vi "TestStand_Go to Temperature Setpoint.vi"(5 "Soak (s)":u32=180, 7 "Timeout (s)":u32=120, 9 "PID Parameters":T1={"Proportional"=0.05, "Integral"=0.0005, "Differential"=-0.0005}, 10 "Tolerance":dbl=0.25 format="%.2f", 11 "Temperature Target":dbl=37.5 caption="Target" format="%.2f") -> (0 "Error Out":errorcluster, 1 "RTD1 Temperature (°C)":dbl=nan format="%.2f", 2 "UUT Temperature (°C)":dbl=nan format="%.2f", 3 "Final Setpoint":dbl=nan format="%.2f", 4 "xPG Charging State":string, 6 "xPG Temperature Level":dbl=nan, 8 "IPG_ReceivedLevel":dbl=nan)   [LabVIEW 2010]
uses:
  Calculations/Temperature Setpoint States.ctl
  <vilib>/ptbypt/NI_PtbyPt.lvlib
panel:
  out "Raw Corrected Temp (°C)":dbl
  in  "stop":bool
  out "Temperature and Delta History":T2(graph)
  out "Setpoint (°C)":dbl=nan format="%.2g"
  out "Temperature Target (°C)":dbl=nan min=25.0 max=80.0 step=0.1 format="%.2f"
  out "Delta_IPG_Target (°C)":dbl=nan format="%.2f"
  out "Air Temperature (°C)":dbl=nan min=25.0 max=80.0 step=0.1 format="%.2f"
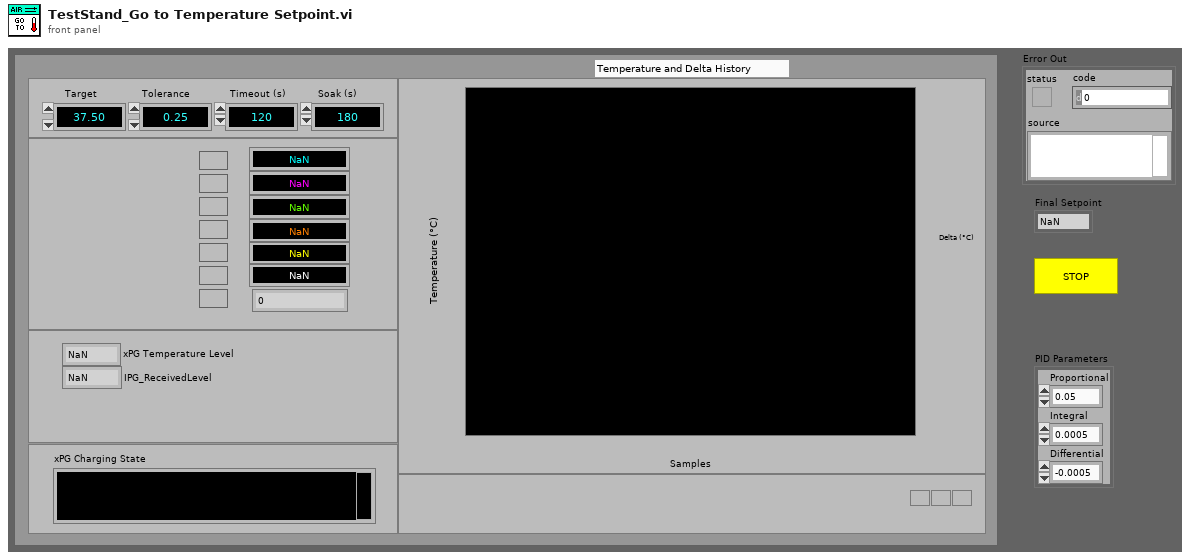
[diagram p1: front panel]
types:
  T1 = cluster{"Proportional":dbl, "Integral":dbl, "Differential":dbl}
  T2 = cluster{"Temperature Target":dbl, "Air Temperature (°C)":dbl, "UUT Temperature (°C)":dbl, "RTD1 Temperature (°C)":dbl, "Setpoint (°C)":dbl, "Delta Setpoint (°C)":dbl, "Delta Setpoint (°C) 2":dbl}
  T3 = cluster{"Temperature Target":dbl, "Air Temperature (°C)":dbl, "UUT Temperature (°C)":dbl, "RTD1 Temperature (°C)":dbl, "Setpoint (°C)":dbl, "Delta Setpoint (°C)":dbl, "Raw Corrected Temp (°C)":dbl}
  T4 = cluster{"Data Index":i32, "Air Blast Ref":refnum<visa-resource-name>, "Tolerance":dbl, "Timeout At":timestamp, "Timed out?":bool, "Previous Millis":u32, "Init PI?":bool, "Soaking?":bool, "Soak Finished At":timestamp, "PID Parameters":cluster{"Proportional":dbl, "Integral":dbl, "Differential":dbl}, "Blast Mode?":bool, "Soak Time (s)":u32, "Init Filter":bool}
  T5 = typedef "Temperature Setpoint States.ctl" = enum16{"Initialize", "Measure", "Update Setpoint", "Update Display", "Check If Done"}
  T6 = cluster{"Temperature Target":dbl, "Air Temperature (°C)":dbl, "UUT Temperature (°C)":dbl, "RTD Temperature (°C)":dbl, "Delta Setpoint (°C)":dbl, "Setpoint (°C)":dbl, "Setpoint (°C) 2":dbl}[]
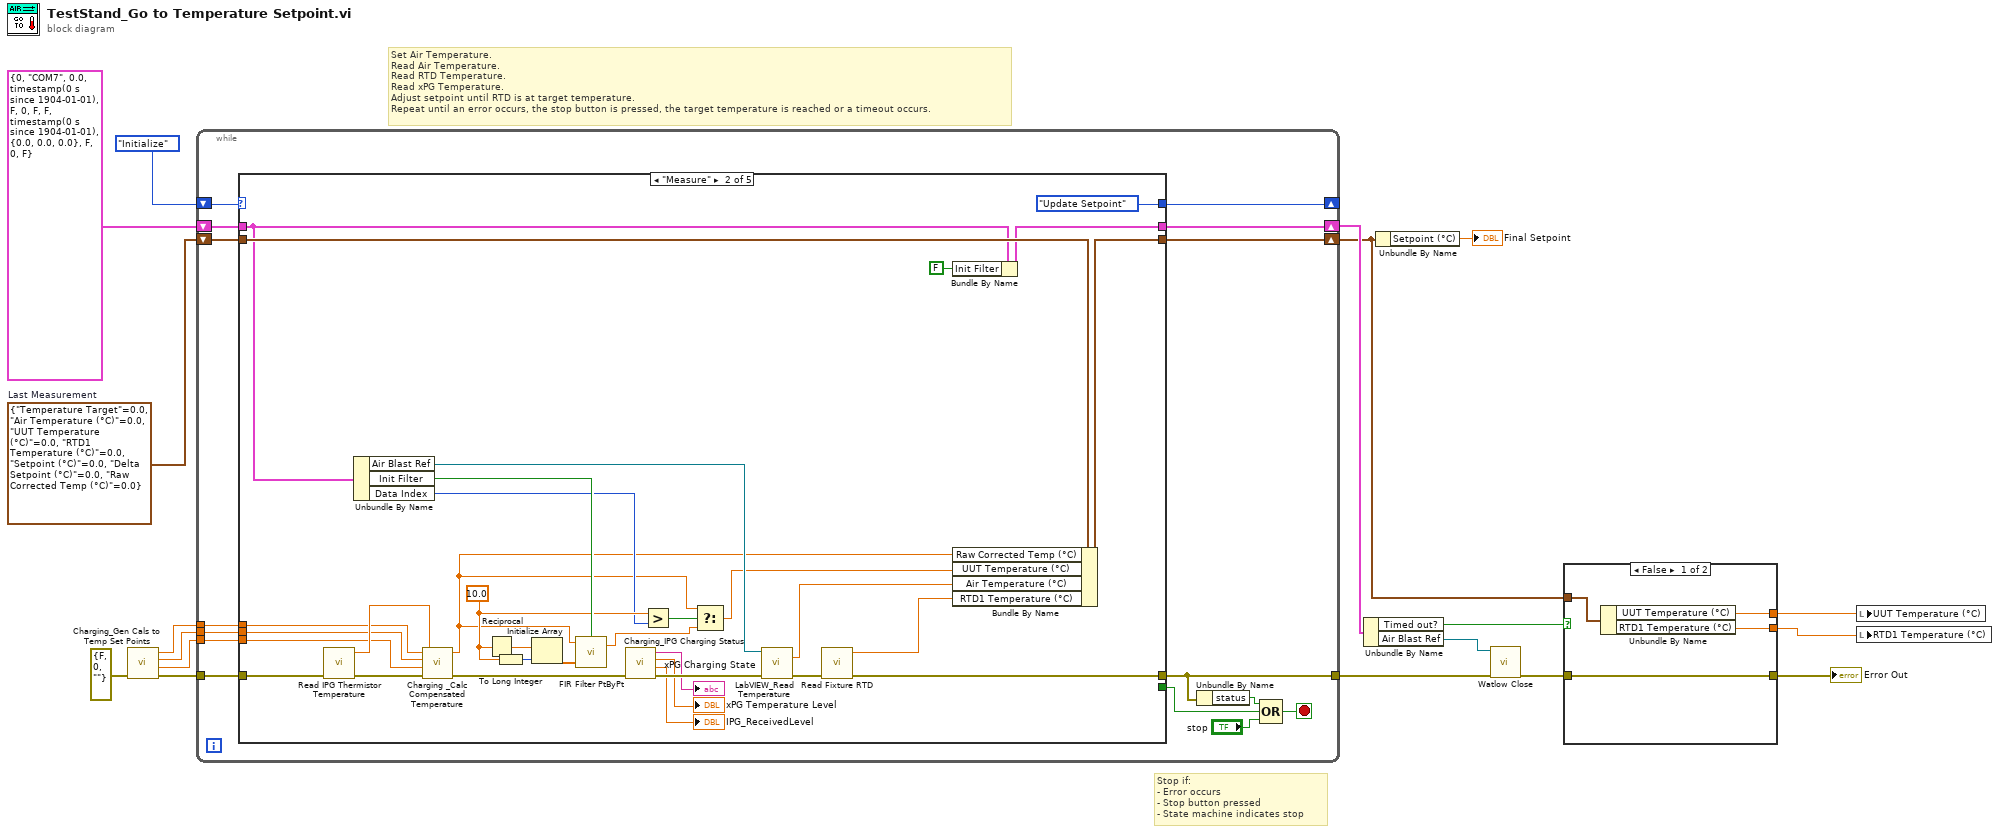
[diagram p0: block diagram]
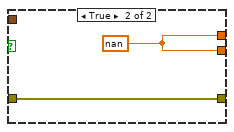
[diagram p2: hidden frame]
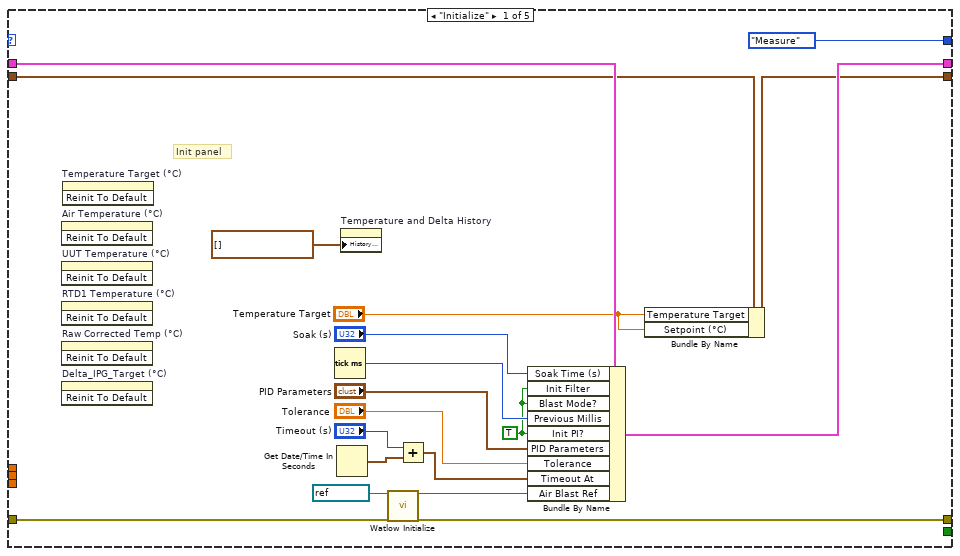
[diagram p3: hidden frame]
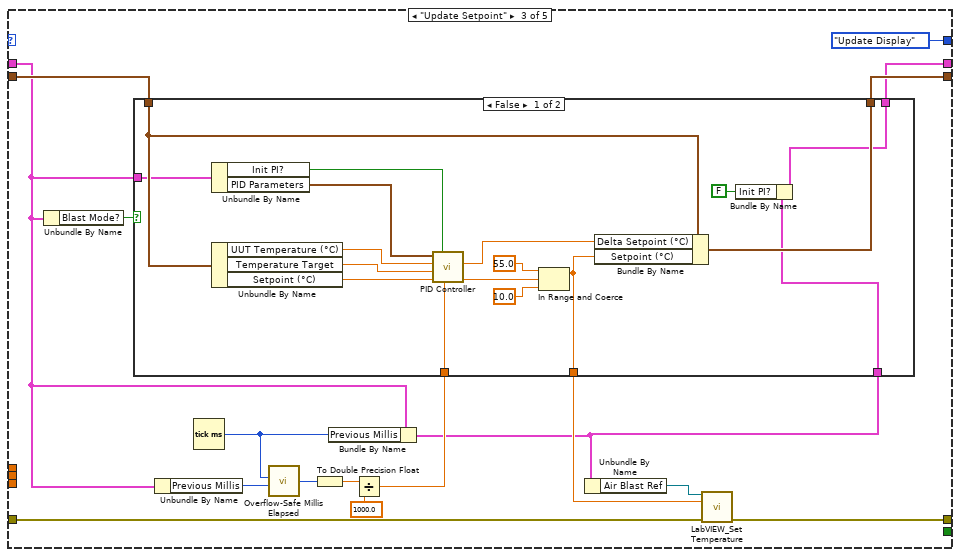
[diagram p4: hidden frame]
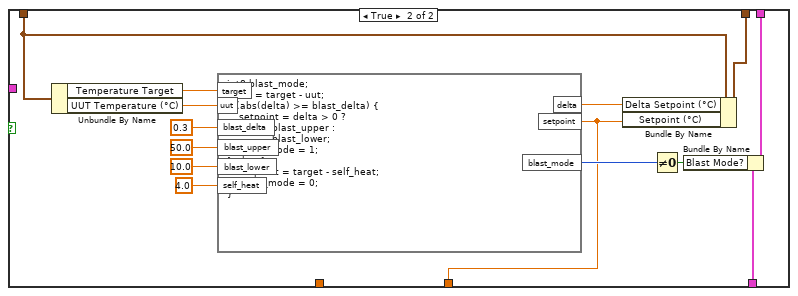
[diagram p5: hidden frame]
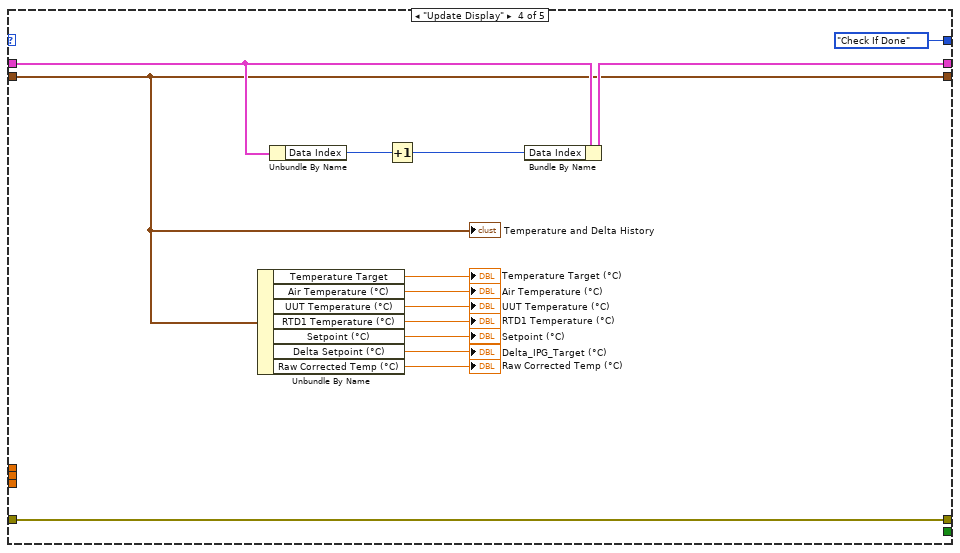
[diagram p6: hidden frame]
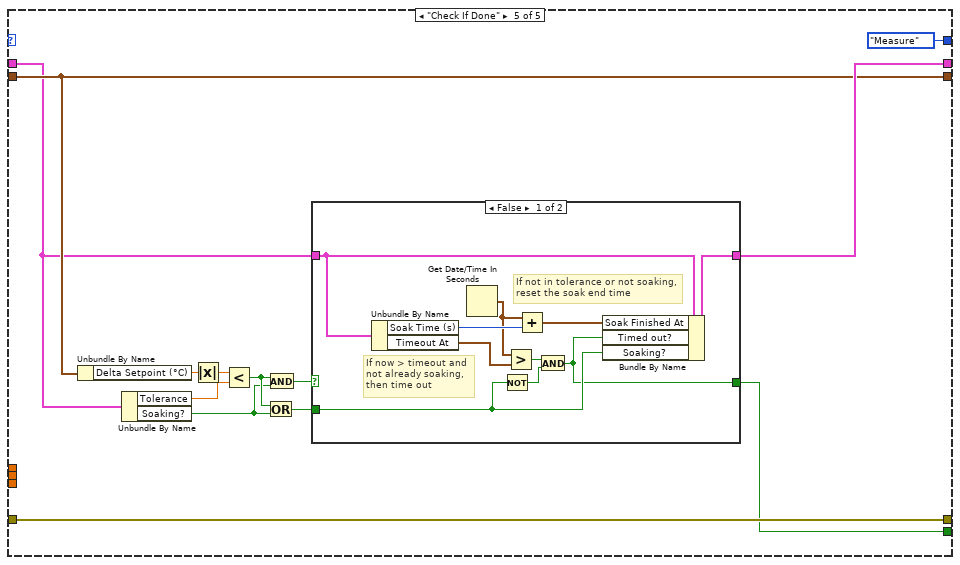
[diagram p7: hidden frame]
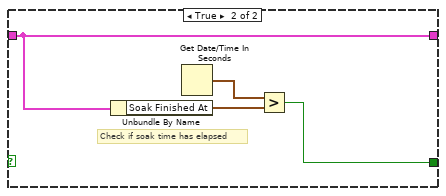
[diagram p8: hidden frame]
diagram:
  w16 = T3 {"Temperature Target"=0.0, "Air Temperature (°C)"=0.0, "UUT Temperature (°C)"=0.0, "RTD1 Temperature (°C)"=0.0, "Setpoint (°C)"=0.0, "Delta Setpoint (°C)"=0.0, "Raw Corrected Temp (°C)"=0.0}  # Last Measurement
  # "Set Air Temperature.\nRead Air Temperature.\nRead RTD Temperature.\nRead xPG Temperature.\nAdjust setpoint until RTD is at target temperature.\nRepeat until an error occurs, the stop button is pressed, the target temperature is reached or a timeout occurs."
  # "Stop if:\n- Error occurs\n- Stop button pressed\n- State machine indicates stop"
  n1 = call "Charging_Gen Cals to Temp Set Points.vi"("error in"=errorcluster {"status"=FALSE, "code"=0, "source"=""} ("Error Out")) -> ("error out"=w10:errorcluster, "Abort Threshold (C)"=w7:dbl, "Critical Threshold (C)"=w8:dbl, "Warning Threshold (C)"=w9:dbl)  [unwired: 6 in, 1 out]
  n2 = while {
    shift-right: [w22] -> _
    shift-left: Temperature_Setpoint_States."Initialize" ("Temperature Setpoint States") -> [w33]
    shift-right: [w32] -> w13
    shift-left: T4 {"Data Index"=0, "Air Blast Ref"="COM7", "Tolerance"=0.0, "Timeout At"=timestamp(0 s since 1904-01-01), "Timed out?"=FALSE, "Previous Millis"=0, "Init PI?"=FALSE, "Soaking?"=FALSE, "Soak Finished At"=timestamp(0 s since 1904-01-01), "PID Parameters"={"Proportional"=0.0, "Integral"=0.0, "Differential"=0.0}, "Blast Mode?"=FALSE, "Soak Time (s)"=0, "Init Filter"=FALSE} -> [w31]
    shift-right: [w23] -> w3
    shift-left: w16 -> [w30]
    tunnel: [w27] -> w14
    tunnel: w10 -> [w29]
    tunnel: w9 -> [w21]
    tunnel: w8 -> [w20]
    tunnel: w7 -> [w19]
    stop <- w28 stop-if-true
    n3 = case shown="\"Measure\"" w33 {
      tunnel: [_ _ _ _ w156] -> w25
      tunnel: [Temperature_Setpoint_States."Measure" ("Temperature Setpoint States") Temperature_Setpoint_States."Update Setpoint" ("Temperature Setpoint States") Temperature_Setpoint_States."Update Display" ("Temperature Setpoint States") Temperature_Setpoint_States."Check If Done" ("Temperature Setpoint States") Temperature_Setpoint_States."Measure" ("Temperature Setpoint States")] -> w22
      tunnel: [w48 w65 w86 w143 w157] -> w32
      tunnel: w31 -> [w50 w66 w88 w145 w151]
      tunnel: w30 -> [w40 w80 w95 w134 w152]
      tunnel: w29 -> [w46 w83 w94 w138 w159]
      tunnel: [w45 w77 w90 w138 w159] -> w27
      tunnel: [w39 w78 w91 w134 w152] -> w23
      tunnel: w21 -> [_ w73 _ _ _]
      tunnel: w20 -> [_ w72 _ _ _]
      tunnel: w19 -> [_ w71 _ _ _]
      frame "Initialize" {
        w35 = TRUE ("Init PID?")
        # "Init panel"
        n4 = invoke on="Air Temperature (°C)" class="DigNum (strict)" method="Reinit To Default"() -> ()  [unwired: 3 in, 3 out]
        n5 = invoke on="UUT Temperature (°C)" class="DigNum (strict)" method="Reinit To Default"() -> ()  [unwired: 3 in, 3 out]
        n6 = invoke on="RTD1 Temperature (°C)" class="DigNum (strict)" method="Reinit To Default"() -> ()  [unwired: 3 in, 3 out]
        n7 = invoke on="Raw Corrected Temp (°C)" class="DigNum (strict)" method="Reinit To Default"() -> ()  [unwired: 3 in, 3 out]
        n8 = invoke on="Delta_IPG_Target (°C)" class="DigNum (strict)" method="Reinit To Default"() -> ()  [unwired: 3 in, 3 out]
        n9 = invoke on="Temperature Target (°C)" class="DigNum (strict)" method="Reinit To Default"() -> ()  [unwired: 3 in, 3 out]
        n10 = Tick Count (ms)() -> (millisecond timer value=w37:u32)
        n11 = Get Date/Time In Seconds() -> (seconds since 1Jan1904=w47:timestamp)
        n12 = property on="Temperature and Delta History" class="WFChart (strict)"("History Data"=T6 []) -> ()  [unwired: 2 in, 2 out]
        n13 = call <instrlib>:"Watlow Initialize.vi"("Comms Port"=refnum<visa-resource-name> "COM7", "Error In"=w46) -> ("UUT Port 2"=w49:refnum<visa-resource-name>, "Error Out"=w45:errorcluster)  [unwired: 16 out]
        n14 = Add(x="Timeout (s)", y=w47) -> (x+y=w43:timestamp)
        n15 = Bundle By Name(cluster=w50, "Soak Time (s)"="Soak (s)", "Init Filter"=w35, "Blast Mode?"=w35, "Previous Millis"=w37, "Init PI?"=w35, "PID Parameters"="PID Parameters", "Tolerance"="Tolerance", "Timeout At"=w43, "Air Blast Ref"=w49) -> (w48:T4)
        n16 = Bundle By Name(cluster=w40, "Temperature Target"="Temperature Target", "Setpoint (°C)"="Temperature Target") -> (w39:T3)
      }
      frame "Measure" {
        w63 = 10.0
        n17 = call "Read IPG Thermistor Temperature.vi"("error in"=w83) -> ("error out"=w74:errorcluster, "Compensated Temperature (C)"=w75:dbl)  [unwired: 7 in, 2 out]
        n18 = Unbundle By Name(w66) -> ("Air Blast Ref"=w82:refnum<visa-resource-name>, "Init Filter"=w67:bool, "Data Index"=w59:i32)
        n19 = call "Charging _Calc Compensated Temperature.vi"("target temperature (C)"=w75, "error in"=w74, "Abort Threshold (42 C)"=w71, "Critical Threshold (41 C)"=w72, "Warning Threshold (40 C)"=w73) -> ("error out"=w58:errorcluster, "compensated temperature (C)"=w53:dbl)  [unwired: 2 in, 1 out]
        n20 = Reciprocal(x=w63) -> (1/x=w70:dbl)
        n21 = To Long Integer(number=w63) -> (32bit integer=w69:i32)
        n22 = Initialize Array(w70, w69) -> (w68:dbl[])
        n23 = call <vilib>:"FIR Filter PtByPt.vi"("initialize"=w67, "Forward Coefficients"=w68, "x"=w53) -> ("Filtered x"=w60:dbl)  [unwired: 1 in, 1 out]
        n24 = call "Charging_IPG Charging Status.vi"("error in"=w58) -> ("error out"=w57:errorcluster, "IPG_ReceivedLevel"=→"IPG_ReceivedLevel":dbl, "TemperatureLevel"=→"xPG Temperature Level":dbl, "ChargingState"=→"xPG Charging State":string)  [unwired: 7 in]
        n25 = Greater?(x=w63, y=w59) -> (0:w62:bool)
        n26 = Select(t=w53, s=w62, f=w60) -> (s? t:f=w61:dbl)
        n27 = call "LabVIEW_Read Temperature.vi"("PC Comms Port"=w82, "error in (no error)"=w57) -> ("Air Temperature (°C)"=w81:dbl, "error out"=w84:errorcluster)  [unwired: 11 in, 1 out]
        n28 = call "Read Fixture RTD.vi"("error in (no error)"=w84) -> ("error out"=w77:errorcluster, "Mean Temperature (C)"=w79:dbl)  [unwired: 7 in, 1 out]
        n29 = Bundle By Name(cluster=w66, "Init Filter"=FALSE) -> (w65:T4)
        n30 = Bundle By Name(cluster=w80, "Raw Corrected Temp (°C)"=w53, "UUT Temperature (°C)"=w61, "Air Temperature (°C)"=w81, "RTD1 Temperature (°C)"=w79) -> (w78:T3)
      }
      frame "Update Setpoint" {
        n31 = Unbundle By Name(w88) -> ("Blast Mode?"=w87:bool)
        n32 = Unbundle By Name(w88) -> ("Previous Millis"=w98:u32)
        n33 = Tick Count (ms)() -> (millisecond timer value=w97:u32)
        n34 = call "Overflow-Safe Millis Elapsed.vi"("now"=w97, "previous"=w98) -> ("elapsed"=w101:u32)  [unwired: 5 in]
        n35 = To Double Precision Float(number=w101) -> (double precision float=w99:dbl)
        n36 = Bundle By Name(cluster=w88, "Previous Millis"=w97) -> (w85:T4)
        n37 = Divide(x=w99, y=1000.0) -> (x/y=w96:dbl)
        n38 = case shown="False" w87 {
          tunnel: w96 -> [w118 _]
          tunnel: w95 -> [w117 w121]
          tunnel: [w116 w119] -> w93
          tunnel: [w115 w120] -> w91
          tunnel: w88 -> [w107 _]
          tunnel: [w103 w131] -> w86
          tunnel: w85 -> [w102 w132]
          frame False {
            n39 = Unbundle By Name(w107) -> ("Init PI?"=w106:bool, "PID Parameters"=w105:T1)
            n40 = Unbundle By Name(w117) -> ("UUT Temperature (°C)"=w109:dbl, "Temperature Target"=w110:dbl, "Setpoint (°C)"=w111:dbl)
            n41 = call "PID Controller.vi"("dt"=w118, "Initialize"=w106, "Previous Set Point"=w111, "Desired Setpoint"=w110, "Measured"=w109, "PID Parameters"=w105) -> ("New Setpoint"=w112:dbl, "Error"=w108:dbl)  [unwired: 4 in]
            n42 = In Range and Coerce(upper limit=55.0 ("y"), x=w112, lower limit=10.0 ("y")) -> (coerced(x)=w116:dbl)  [unwired: 1 out]
            n43 = Bundle By Name(cluster=w117, "Delta Setpoint (°C)"=w108, "Setpoint (°C)"=w116) -> (w115:T3)
            n44 = Bundle By Name(cluster=w102, "Init PI?"=FALSE) -> (w103:T4)
          }
          frame True {
            n45 = Unbundle By Name(w121) -> ("Temperature Target"=w128:dbl, "UUT Temperature (°C)"=w127:dbl)
            n46 = formula code="int8 blast_mode;\ndelta = target - uut;\nif (abs(delta) >= blast_delta) {\n    setpoint = delta > 0 ? \n               blast_upper :\n               blast_lower;\n    blast_mode = 1;\n} else {\n    setpoint = target - self_heat;\n    blast_mode = 0;\n}"("target"=w128, "uut"=w127, "self_heat"=4.0 ("input variable"), "blast_delta"=0.3 ("input variable"), "blast_upper"=50.0 ("input variable"), "blast_lower"=10.0 ("input variable")) -> ("delta"=w122:dbl, "setpoint"=w119:dbl, "blast_mode"=w130:i8)
            n47 = Bundle By Name(cluster=w121, "Delta Setpoint (°C)"=w122, "Setpoint (°C)"=w119) -> (w120:T3)
            n48 = Not Equal To 0?(x=w130) -> (x != 0?=w129:bool)
            n49 = Bundle By Name(cluster=w132, "Blast Mode?"=w129) -> (w131:T4)
          }
        }
        n50 = Unbundle By Name(w85) -> ("Air Blast Ref"=w92:refnum<visa-resource-name>)
        n51 = call "LabVIEW_Set Temperature.vi"("PC Comms Port"=w92, "Air Temperature Setpoint (°C)"=w93, "error in (no error)"=w94) -> ("error out"=w90:errorcluster)  [unwired: 11 in, 1 out]
      }
      frame "Update Display" {
        n52 = Unbundle By Name(w134) -> ("Temperature Target"=→"Temperature Target (°C)":dbl, "Air Temperature (°C)"=→"Air Temperature (°C)":dbl, "UUT Temperature (°C)"=→"UUT Temperature (°C)":dbl, "RTD1 Temperature (°C)"=→"RTD1 Temperature (°C)":dbl, "Setpoint (°C)"=→"Setpoint (°C)":dbl, "Delta Setpoint (°C)"=→"Delta_IPG_Target (°C)":dbl, "Raw Corrected Temp (°C)"=→"Raw Corrected Temp (°C)":dbl)
        n53 = Unbundle By Name(w145) -> ("Data Index"=w146:i32)
        n54 = Increment(x=w146) -> (x+1=w144:i32)
        n55 = Bundle By Name(cluster=w145, "Data Index"=w144) -> (w143:T4)
        "Temperature and Delta History" <- w134
      }
      frame "Check If Done" {
        n56 = Unbundle By Name(w152) -> ("Delta Setpoint (°C)"=w153:dbl)
        n57 = Unbundle By Name(w151) -> ("Tolerance"=w154:dbl, "Soaking?"=w147:bool)
        n58 = Absolute Value(x=w153) -> (abs(x)=w155:dbl)
        n59 = Less?(x=w155, y=w154) -> (x < y?=w149:bool)
        n60 = Or(x=w149, y=w147) -> (x .or. y?=w148:bool)
        n61 = And(x=w149, y=w147) -> (x .and. y?=w150:bool)
        n62 = case shown="False" w150 {
          tunnel: [w161 w171] -> w156
          tunnel: [w160 w170] -> w157
          tunnel: w151 -> [w167 w170]
          tunnel: w148 -> [w162 _]
          frame False {
            # "If now > timeout and not already soaking, then time out"
            # "If not in tolerance or not soaking, reset the soak end time"
            n63 = Unbundle By Name(w167) -> ("Soak Time (s)"=w168:u32, "Timeout At"=w165:timestamp)
            n64 = Get Date/Time In Seconds() -> (seconds since 1Jan1904=w166:timestamp)
            n65 = Not(x=w162) -> (.not. x?=w163:bool)
            n66 = Greater?(x=w166, y=w165) -> (0:w164:bool)
            n67 = Add(x=w166, y=w168) -> (x+y=w169:timestamp)
            n68 = And(x=w164, y=w163) -> (x .and. y?=w161:bool)
            n69 = Bundle By Name(cluster=w167, "Soak Finished At"=w169, "Timed out?"=w161, "Soaking?"=w162) -> (w160:T4)
          }
          frame True {
            # "Check if soak time has elapsed"
            n70 = Unbundle By Name(w170) -> ("Soak Finished At"=w172:timestamp)
            n71 = Get Date/Time In Seconds() -> (seconds since 1Jan1904=w173:timestamp)
            n72 = Greater?(x=w173, y=w172) -> (0:w171:bool)
          }
        }
      }
    }
    n73 = Unbundle By Name(w27) -> ("status"=w26:bool)
    n74 = Compound Arithmetic op=OR(w26, w25, "stop") -> (w28:bool)
  }
  n75 = Unbundle By Name(w13) -> ("Timed out?"=w6:bool, "Air Blast Ref"=w15:refnum<visa-resource-name>)
  n76 = Unbundle By Name(w3) -> ("Setpoint (°C)"=→"Final Setpoint":dbl)
  n77 = call <instrlib>:"Watlow Close.vi"("PC Comms Port"=w15, "Error In"=w14) -> ("Error Out"=w5:errorcluster)  [unwired: 16 in, 1 out]
  n78 = case shown="False" w6 {
    tunnel: w5 -> [w177 w178]
    tunnel: [w177 w178] -> w4
    tunnel: w3 -> [w174 _]
    tunnel: [w176 w179] -> w2
    tunnel: [w175 w179] -> w1
    frame False {
      n79 = Unbundle By Name(w174) -> ("UUT Temperature (°C)"=w176:dbl, "RTD1 Temperature (°C)"=w175:dbl)
    }
    frame True {
      w179 = nan
    }
  }
  "Error Out" <- w4
  n80 = local write "UUT Temperature (°C)"(w2) -> ()
  n81 = local write "RTD1 Temperature (°C)"(w1) -> ()
